vi "Set Self Attributes.vi"(10 "Self Attributes":refnum<class "Attributes.lvclass">, 11 "Sender in":refnum<class "Sender.lvclass">) -> (3 "Sender out":refnum<class "Sender.lvclass">)   [LabVIEW 2020, in "jettl.lvlib" / "Sender.lvlib" / "Sender.lvclass"]
uses:
  Sender.lvclass
  Attributes/Attributes/Attributes.lvclass
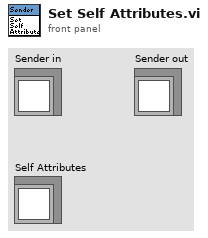
[diagram p1: front panel]
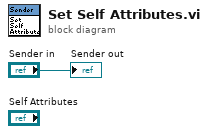
[diagram p0: block diagram]
diagram:
  "Sender out" <- "Sender in"
